vi "fourier decomposition.vi"() -> ()   [LabVIEW 2020]
uses:
  <vilib>/measure/matone.llb/Extract Single Tone Information 1 Chan.vi
  <vilib>/express/express analysis/Spectral/Block/exnSpectralBlock spectral measurements RMS poly.vi
  <vilib>/express/express analysis/Spectral/Block/exnSpectralBlock spectral measurements RMS WFM.vi
  <vilib>/express/express analysis/Spectral/XNode/ExpressSpectralMeasurementsBlockNode.xnode
  <vilib>/measure/NI_MABase.lvlib
  <vilib>/measure/NI_MAPro.lvlib
panel:
  out "fft":cluster{"f0":dbl, "df":dbl, "magnitude":dbl[]}(graph)
  out "Waveform Graph":dynamicdata(graph)
  in  "harminoc5":bool
  in  "harminoc3":bool
  in  "N":dbl=1.0 format="%0.2p"
  in  "fs":dbl=1.0 format="%0.2p"
  in  "signal type":T1(ring)
  in  "frequency":dbl=10.0 format="%0.2p"
  in  "amplitude":dbl=1.0 format="%0.2p"
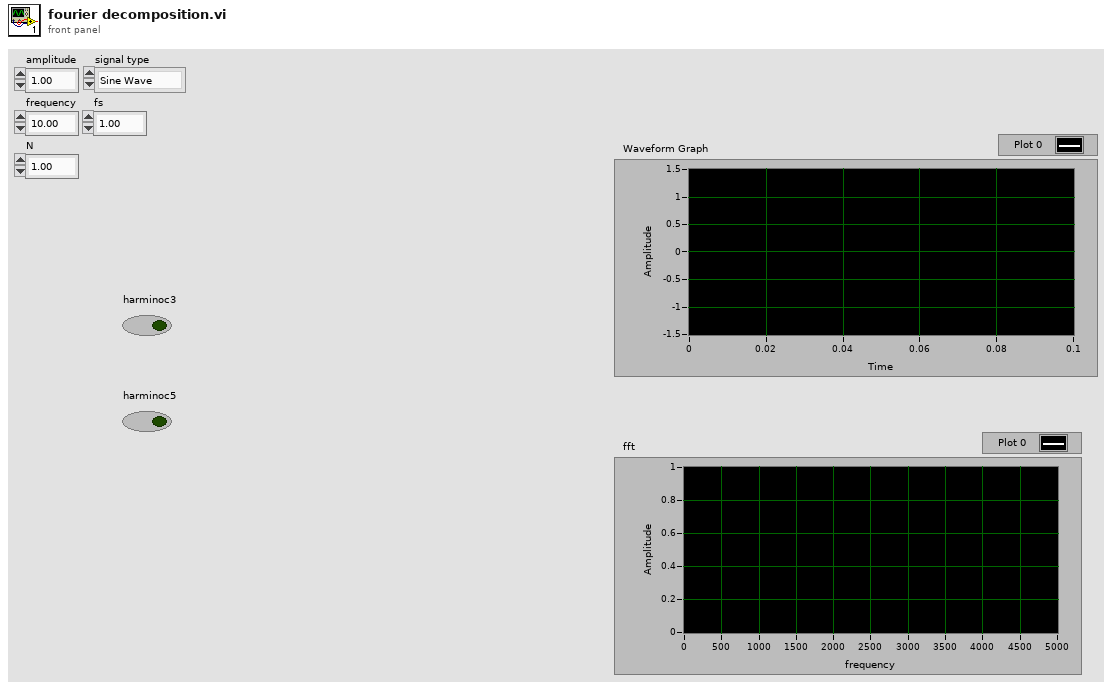
[diagram p1: front panel]
types:
  T1 = enum16{"Sine Wave", "Triangle Wave", "Square Wave", "Sawtooth Wave"}
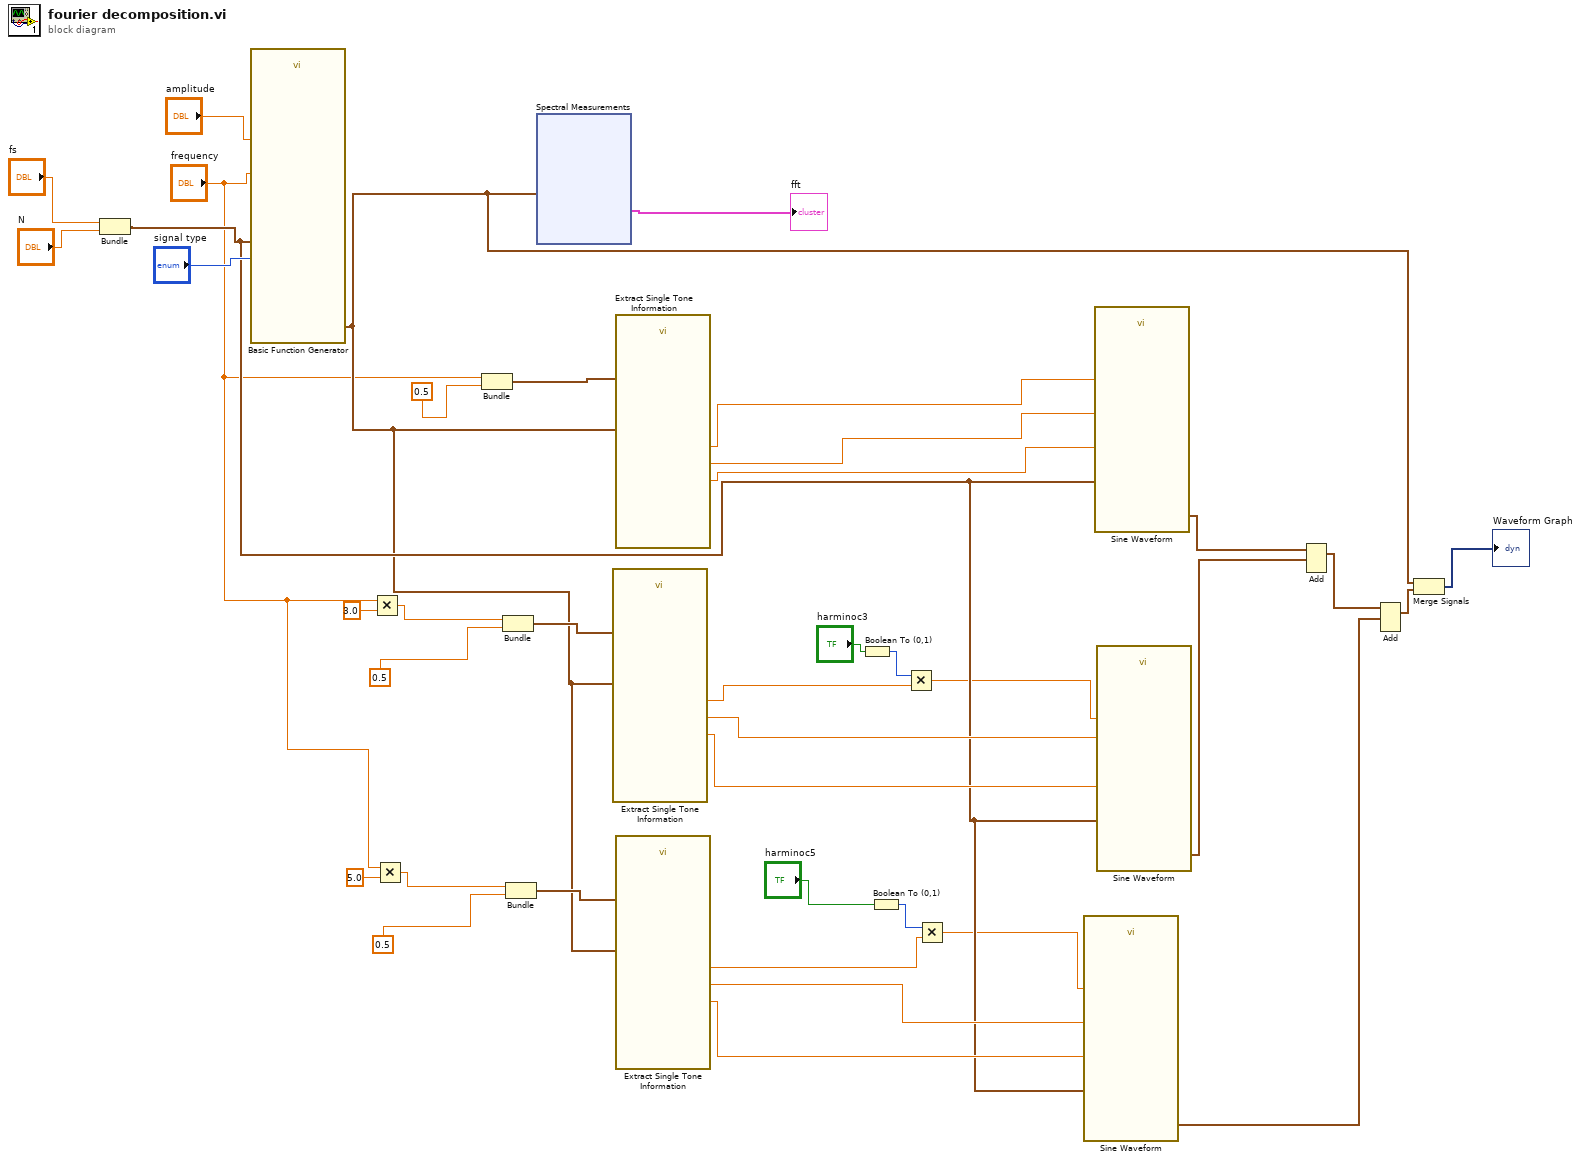
[diagram p0: block diagram]
diagram:
  n1 = Bundle("fs"="fs", "N"="N") -> (w18:cluster{"fs":dbl, "N":dbl})  [unwired: 1 in]
  n2 = call <vilib>:"Basic Function Generator.vi"("sampling info"=w18, "signal type"="signal type", "amplitude"="amplitude", "frequency"="frequency") -> ("signal out"=w3:waveform(dbl))  [unwired: 5 in, 2 out]
  n3 = Multiply(x="frequency", y=3.0) -> (x*y=w31:dbl)
  n4 = Multiply(x="frequency", y=5.0) -> (x*y=w27:dbl)
  n5 = Bundle("frequency"="frequency", 0.5) -> (w34:cluster{"frequency":dbl, dbl})  [unwired: 1 in]
  n6 = Bundle(w31, 0.5) -> (w32:cluster{dbl, dbl})  [unwired: 1 in]
  n7 = Bundle(w27, 0.5) -> (w28:cluster{dbl, dbl})  [unwired: 1 in]
  n8 = xnode "Spectral Measurements"("Signals"=w3) -> ("FFT - (RMS)"=→"fft":cluster{"f0":dbl, "df":dbl, "magnitude":dbl[]})  [unwired: 1 in, 2 out]
  n9 = call-poly <vilib>:"Extract Single Tone Information.vi"("advanced search"=w32, "time signal in"=w3) -> ("detected phase (deg)"=w21:dbl, "detected amplitude"=w14:dbl, "detected frequency"=w22:dbl)  [unwired: 4 in, 3 out]
  n10 = call-poly <vilib>:"Extract Single Tone Information.vi"("advanced search"=w34, "time signal in"=w3) -> ("detected phase (deg)"=w23:dbl, "detected amplitude"=w25:dbl, "detected frequency"=w24:dbl)  [unwired: 4 in, 3 out]
  n11 = call-poly <vilib>:"Extract Single Tone Information.vi"("advanced search"=w28, "time signal in"=w3) -> ("detected phase (deg)"=w19:dbl, "detected amplitude"=w12:dbl, "detected frequency"=w20:dbl)  [unwired: 4 in, 3 out]
  n12 = Boolean To (0,1)(Boolean="harminoc3") -> (0, 1=w15:i16)
  n13 = Boolean To (0,1)(Boolean="harminoc5") -> (0, 1=w11:i16)
  n14 = Multiply(x=w15, y=w14) -> (x*y=w13:dbl)
  n15 = Multiply(x=w11, y=w12) -> (x*y=w10:dbl)
  n16 = call <vilib>:"Sine Waveform.vi"("sampling info"=w18, "phase"=w19, "amplitude"=w10, "frequency"=w20) -> ("signal out"=w6:waveform(dbl))  [unwired: 6 in, 1 out]
  n17 = call <vilib>:"Sine Waveform.vi"("sampling info"=w18, "phase"=w23, "amplitude"=w25, "frequency"=w24) -> ("signal out"=w8:waveform(dbl))  [unwired: 6 in, 1 out]
  n18 = call <vilib>:"Sine Waveform.vi"("sampling info"=w18, "phase"=w21, "amplitude"=w13, "frequency"=w22) -> ("signal out"=w7:waveform(dbl))  [unwired: 6 in, 1 out]
  n19 = Add(1:w7, 2:w8) -> (0:w5:waveform(dbl))  [unwired: 1 in, 1 out]
  n20 = Add(1:w6, 2:w5) -> (0:w4:waveform(dbl))  [unwired: 1 in, 1 out]
  n21 = Merge Signals(w3, w4) -> (→"Waveform Graph":dynamicdata)
